vi "leernumerospares.vi"() -> ()   [LabVIEW 2011]
panel:
  out "Array":dbl[](array[numeric])
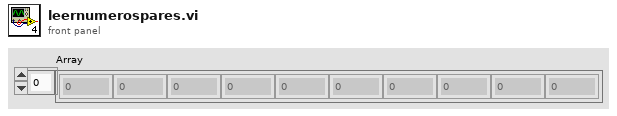
[diagram p1: front panel]
types:
  T1 = enum16{"open", "replace", "create", "open or create", "replace or create", "replace or create with confirmation"}
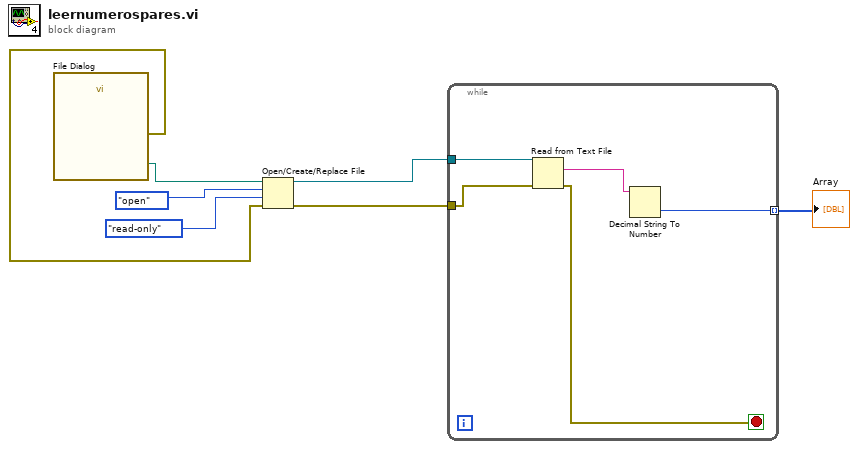
[diagram p0: block diagram]
diagram:
  n1 = call "File Dialog"() -> ("selected path"=w6:path, "error out"=w7:errorcluster)  [unwired: 12 in, 2 out]
  n2 = Open/Create/Replace File(file path (use dialog)=w6, error in=w7, operation (0:open)=T1."open", access (0:read/write)=enum16{"read/write", "read-only", "write-only"}."read-only") -> (refnum out=w3:refnum<file>, error out=w2:errorcluster)  [unwired: 2 in, 1 out]
  n3 = while {
    tunnel: w3 -> [w10]
    tunnel: w2 -> [w11]
    tunnel: [w12] -> w1 mode=indexing
    stop <- w9 stop-if-true
    n4 = Read from Text File(file (use dialog)=w10, error in=w11) -> (text=w8:string, error out=w9:errorcluster)  [unwired: 2 in, 2 out]
    n5 = Decimal String To Number(string=w8) -> (number=w12:i32)  [unwired: 2 in, 1 out]
  }
  "Array" <- w1
